vi "evaluateNestedEmptyElement.vi"(8 "error in (no error)":errorcluster, 9 "a":cluster{"b":cluster{"a":string}}, 10 "XML String":string="<a>\n  <b>\n    <a/>\n  </b>\n</a>", 11 "reference in":refnum<class "EasyXML_XML_Subset_Evaluations.lvclass">) -> (0 "error out":errorcluster, 2 "a":cluster{"b":cluster{"a":string}}, 3 "reference in":refnum<class "EasyXML_XML_Subset_Evaluations.lvclass">)   [LabVIEW 2013, in "EasyXML_XML_Subset_Evaluations.lvclass"]
uses:
  EasyXML_XML_Subset_Evaluations.lvclass
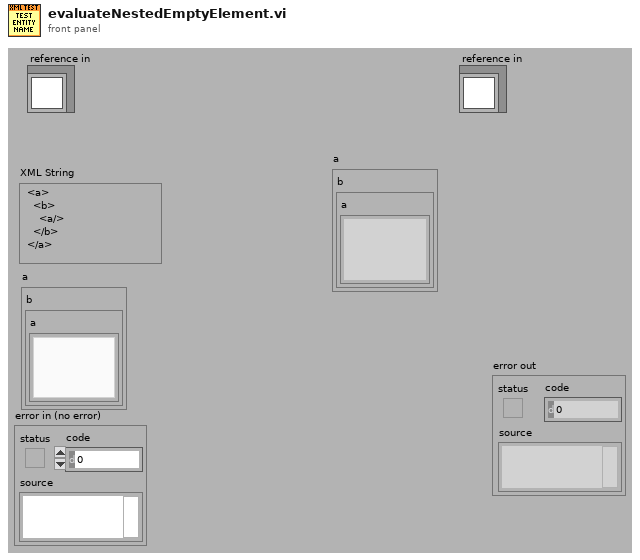
[diagram p1: front panel]
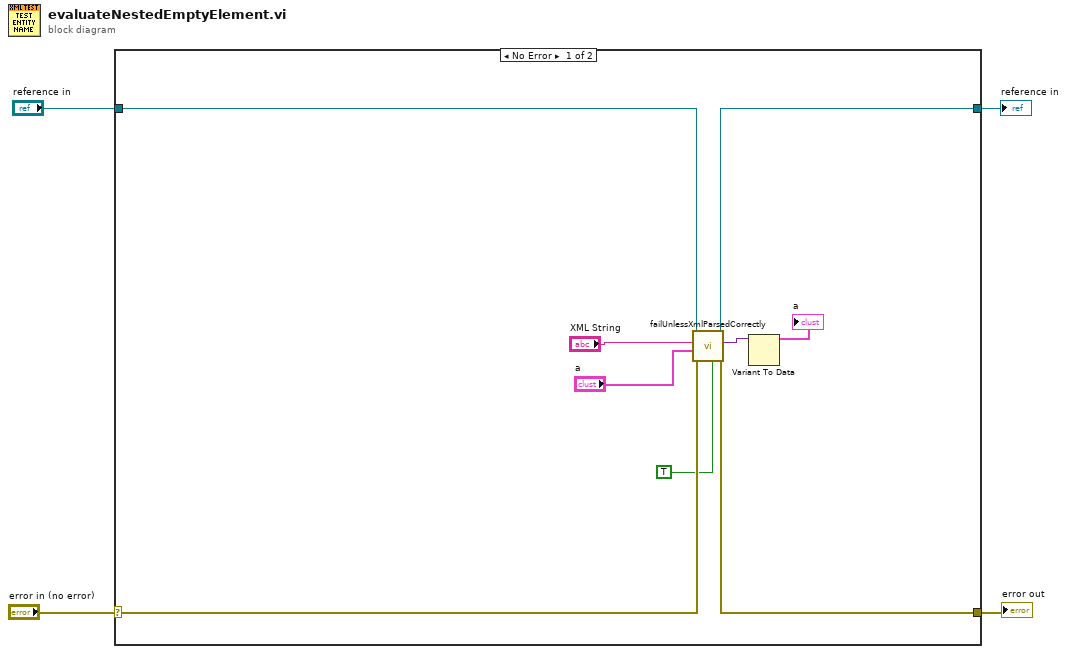
[diagram p0: block diagram]
diagram:
  n1 = case shown="No Error" "error in (no error)" {
    selector: "error in (no error)" -> [w11 w15]
    tunnel: [w6 w15] -> w3
    tunnel: [w12 w14] -> w1
    tunnel: "reference in" -> [w13 w14]
    frame No Error {
      n2 = call "failUnlessXmlParsedCorrectly.vi"("Convert EOL? (TRUE)"=TRUE, "error in"=w11, "Expected Data"="a", "XML String"="XML String", "reference in"=w13) -> ("error out"=w6:errorcluster, "Produced Data"=w9:variant, "reference in"=w12:refnum<class "EasyXML_XML_Subset_Evaluations.lvclass">)  [unwired: 4 in]
      n3 = Variant To Data(Variant=w9) -> (data=→"a":cluster{"b":cluster{"a":string}})  [unwired: 2 in, 1 out]
    }
    frame Error {
    }
  }
  "error out" <- w3
  "reference in" <- w1
